vi "Motor_Meas.vi"(9 "y":i32, 10 "COM":refnum<visa-resource-name> caption="COM\nPort", 11 "error":T1={"status"=FALSE, "code"=1073676294, "source"="VISA Read in MotorBack 2(SubVI).vi->Main_E8361C_2.vi"}) -> (2 "Locat":dbl caption="Current Location" format="%#.1f deg.", 3 "error 2":T1={"status"=FALSE, "code"=1073676294, "source"="VISA Read in MotorBack 2(SubVI).vi->Main_E8361C_2.vi"})   [LabVIEW 2020]
uses:
  D:/weiluntest/visaerror.ctl
  D:/BWant RT/BWant_RT.lvlibp/Control Function.ctl
  D:/BWant RT/BWant_RT.lvlibp
panel:
  out "Boolean":bool
  in  "Stop":bool
  out "[ALM-A]":bool
  in  "Mode":enum16{"INC", "ABS"}(ring)=enum."ABS"
  out "[READY]":bool
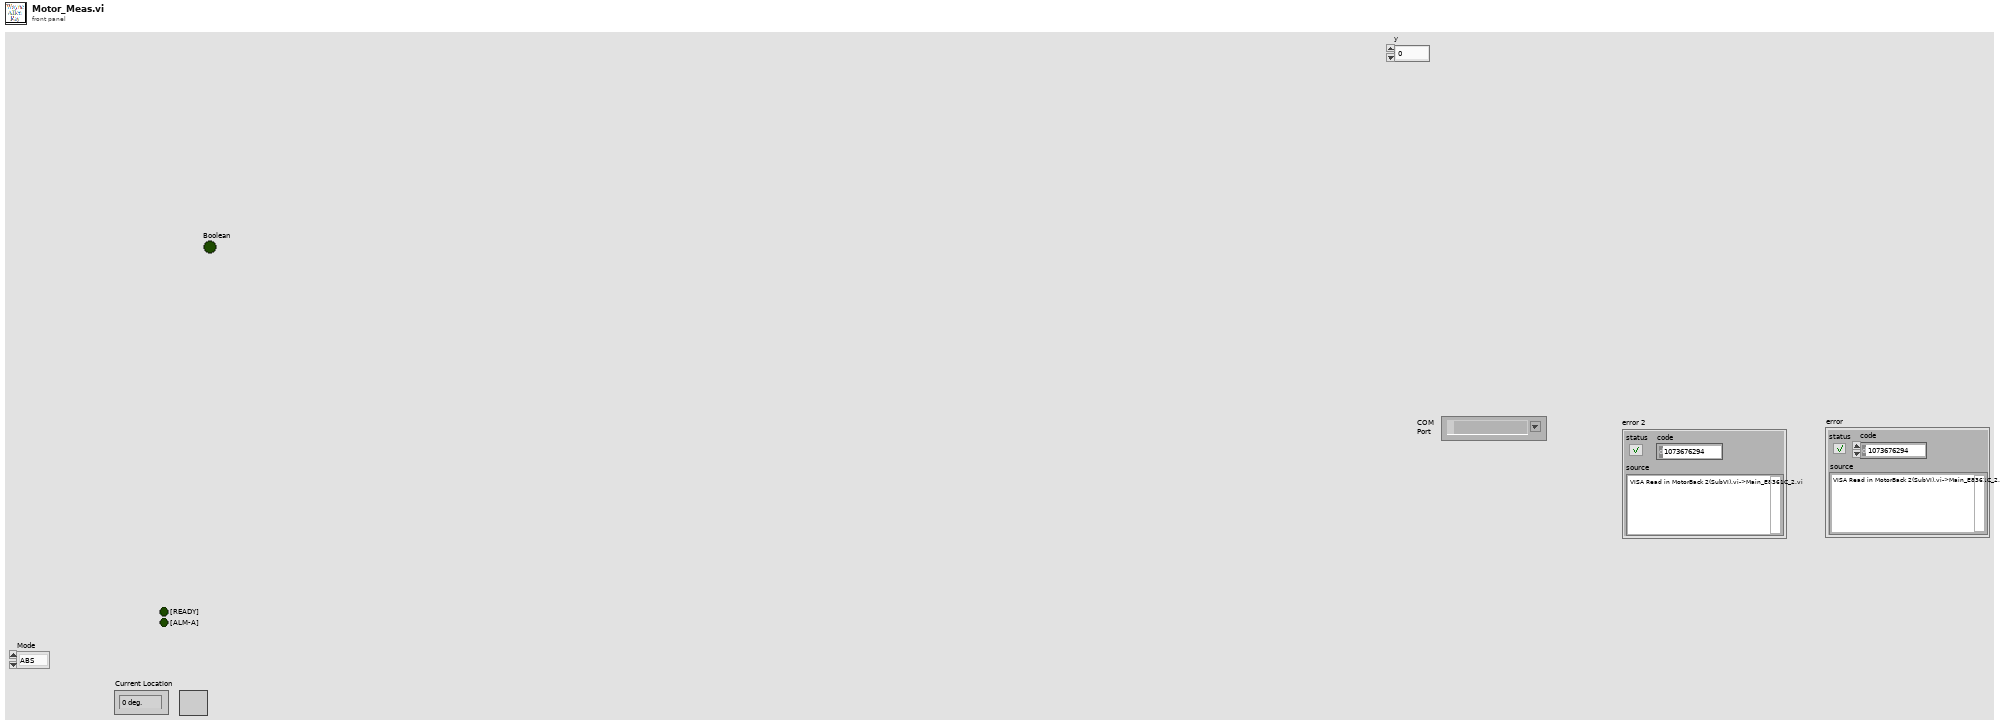
[diagram p1: front panel]
types:
  T1 = typedef "visaerror.ctl" = errorcluster
  T2 = typedef "BWant_RT.lvlibp/Control Function.ctl" = enum16{"Idle", "Initial", "Close", "Check State", "ALM Reset", "ALM Inf", "Preset Home", "Pst_Value", "Speed", "Start-slope", "End-slpoe", "Read Pst", "GO Home", "Move", "Stop", "Limit mode", "MLU", "MLL", "Direction"}
  T3 = cluster{"[MOVE]":bool, "[READY]":bool, "[ALM-A]":bool}
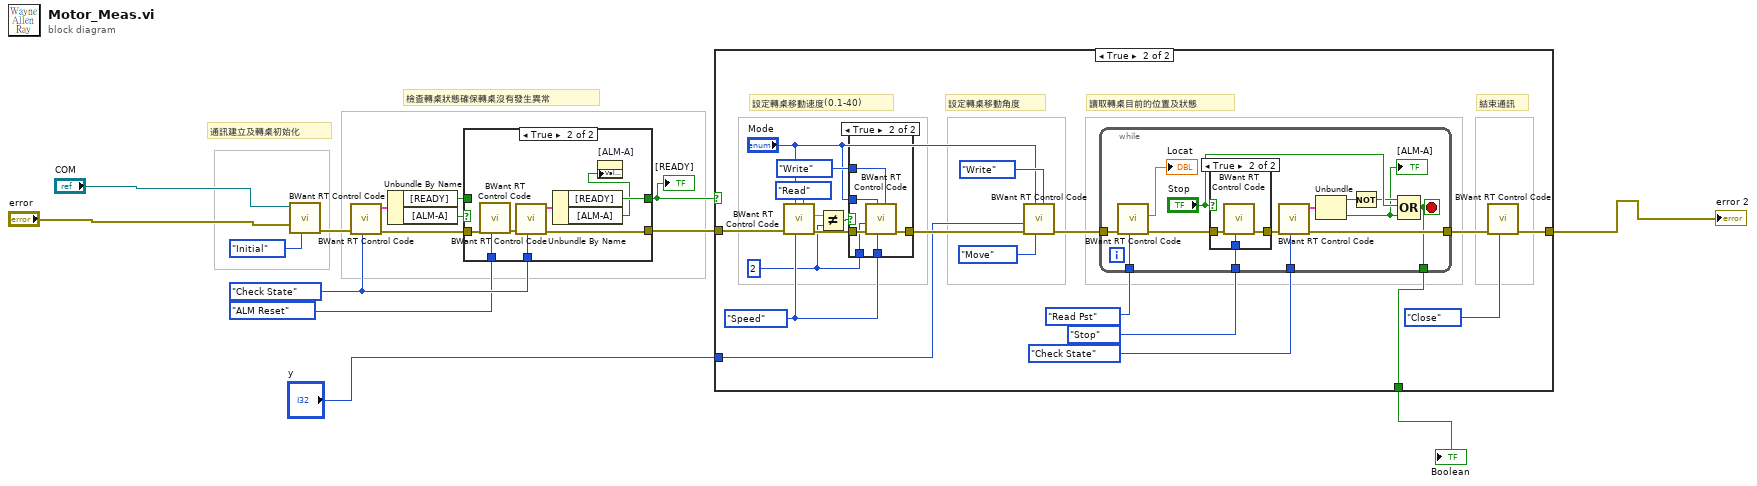
[diagram p0: block diagram]
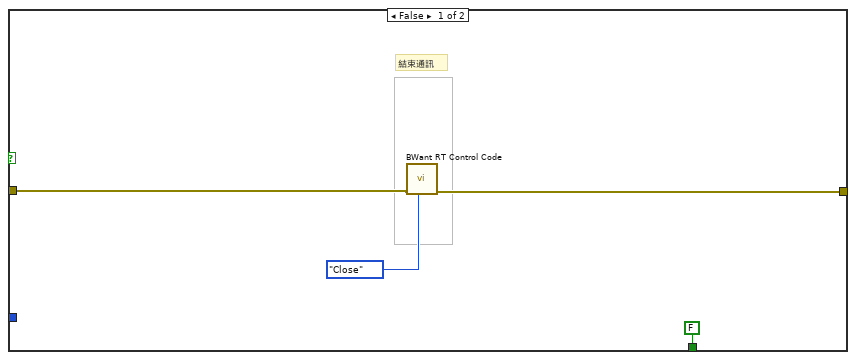
[diagram p2: hidden frame]
diagram:
  w7 = Control_Function."Check State" ("Fn")
  # "檢查轉桌狀態確保轉桌沒有發生異常"
  # "通訊建立及轉桌初始化"
  n1 = call "BWant RT Control Code.vi"("Fn"=Control_Function."Initial", "error in"="error", "ComPort"="COM") -> ("error out"=w12:errorcluster)  [unwired: 5 in, 3 out]
  n2 = call "BWant RT Control Code.vi"("Fn"=w7, "error in"=w12) -> ("error out"=w14:errorcluster, "State"=w13:T3)  [unwired: 6 in, 2 out]
  n3 = Unbundle By Name(w13) -> ("[READY]"=w11:bool, "[ALM-A]"=w15:bool)
  n4 = case shown="True" w15 {
    tunnel: [w17 w23] -> w10
    tunnel: w14 -> [w17 w19]
    tunnel: Control_Function."ALM Reset" ("Fn") -> [_ w25]
    tunnel: w7 -> [_ w22]
    tunnel: [w16 w20] -> w9
    tunnel: w11 -> [w16 _]
    frame False {
    }
    frame True {
      n5 = call "BWant RT Control Code.vi"("Fn"=w25, "error in"=w19) -> ("error out"=w24:errorcluster)  [unwired: 6 in, 3 out]
      n6 = call "BWant RT Control Code.vi"("Fn"=w22, "error in"=w24) -> ("error out"=w23:errorcluster, "State"=w21:T3)  [unwired: 6 in, 2 out]
      n7 = Unbundle By Name(w21) -> ("[READY]"=w20:bool, "[ALM-A]"=w18:bool)
      n8 = property on="[ALM-A]" class="Bool (strict)"("Value"=w18) -> ()  [unwired: 2 in, 2 out]
    }
  }
  "[READY]" <- w9
  n9 = case shown="True" w9 {
    tunnel: w10 -> [w29 w50]
    tunnel: [w28 w40] -> w5
    tunnel: "y" -> [_ w31]
    tunnel: [FALSE w30] -> w1
    frame False {
      # "結束通訊"
      n10 = call "BWant RT Control Code.vi"("Fn"=Control_Function."Close", "error in"=w29) -> ("error out"=w28:errorcluster)  [unwired: 6 in, 3 out]
    }
    frame True {
      w32 = 2
      w38 = Control_Function."Speed" ("Fn")
      # "結束通訊"
      # "讀取轉桌目前的位置及狀態"
      # "設定轉桌移動角度"
      # "設定轉桌移動速度(0.1-40)"
      n11 = call "BWant RT Control Code.vi"("Value_RW"=enum16{"Read", "Write"}."Read", "Fn"=w38, "Mode"="Mode", "error in"=w50) -> ("error out"=w48:errorcluster, "Value out"=w47:dbl)  [unwired: 4 in, 2 out]
      n12 = Not Equal?(x=w47, y=w32) -> (x != y?=w45:bool)
      n13 = case shown="True" w45 {
        tunnel: w48 -> [w69 w75]
        tunnel: w38 -> [_ w74]
        tunnel: w32 -> [_ w73]
        tunnel: enum16{"Read", "Write"}."Write" ("Value_RW") -> [_ w72]
        tunnel: [w69 w71] -> w43
        tunnel: "Mode" -> [_ w70]
        frame False {
        }
        frame True {
          n14 = call "BWant RT Control Code.vi"("Value_RW"=w72, "Fn"=w74, "Mode"=w70, "error in"=w75, "Value in"=w73) -> ("error out"=w71:errorcluster)  [unwired: 3 in, 3 out]
        }
      }
      n15 = call "BWant RT Control Code.vi"("Value_RW"=enum16{"Read", "Write"}."Write", "Fn"=Control_Function."Move", "Mode"="Mode", "error in"=w43, "Value in"=w31) -> ("error out"=w42:errorcluster)  [unwired: 3 in, 3 out]
      n16 = while {
        tunnel: w42 -> [w64]
        tunnel: Control_Function."Read Pst" ("Fn") -> [w63]
        tunnel: Control_Function."Stop" ("Fn") -> [w60]
        tunnel: Control_Function."Check State" ("Fn") -> [w58]
        tunnel: [w56] -> w41
        tunnel: [w51] -> w30
        stop <- w51 stop-if-true
        n17 = call "BWant RT Control Code.vi"("Fn"=w63, "error in"=w64) -> ("error out"=w61:errorcluster, "Value out"=→"Locat":dbl)  [unwired: 6 in, 2 out]
        n18 = case shown="True" "Stop" {
          tunnel: w61 -> [w65 w68]
          tunnel: w60 -> [_ w67]
          tunnel: [w65 w66] -> w59
          frame False {
          }
          frame True {
            n19 = call "BWant RT Control Code.vi"("Fn"=w67, "error in"=w68) -> ("error out"=w66:errorcluster)  [unwired: 6 in, 3 out]
          }
        }
        n20 = call "BWant RT Control Code.vi"("Fn"=w58, "error in"=w59) -> ("error out"=w56:errorcluster, "State"=w57:T3)  [unwired: 6 in, 2 out]
        n21 = Unbundle(w57) -> ("[MOVE]"=w55:bool, "[ALM-A]"=w52:bool)  [unwired: 1 out]
        "[ALM-A]" <- w52
        n22 = Not(x=w55) -> (.not. x?=w53:bool)
        n23 = Compound Arithmetic op=OR(w53, "Stop", w52) -> (w51:bool)
      }
      n24 = call "BWant RT Control Code.vi"("Fn"=Control_Function."Close", "error in"=w41) -> ("error out"=w40:errorcluster)  [unwired: 6 in, 3 out]
    }
  }
  "error 2" <- w5
  "Boolean" <- w1
